vi "onSuiteSlippage.vi"(7 "BananaPeel in":refnum<class "BananaPeel.lvclass">, 11 "Leaf.TestSuite":refnum<class "Leaf.TestSuite.lvclass">) -> (0 "error out":errorcluster, 3 "Leaf.TestSuite":refnum<class "Leaf.TestSuite.lvclass">)   [LabVIEW 2021, in "Bananas.lvlib" / "BananaPeel.lvclass"]
uses:
  BananaPeel.lvclass
  Leaf.TestSuite/Leaf.TestSuite.lvclass
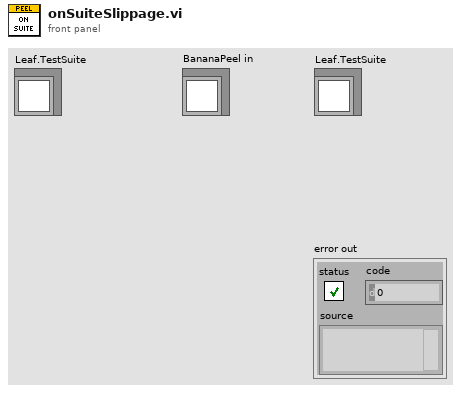
[diagram p1: front panel]
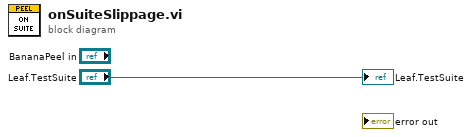
[diagram p0: block diagram]
diagram:
  "Leaf.TestSuite" <- "Leaf.TestSuite"
